vi "Popup Dialog.vi"(5 "Tab Control":T1, 8 "error in (no error)":errorcluster, 9 "show":bool, 10 "Error MSG":string, 11 "Delay (5sec)":dbl=5.0) -> (0 "error out":errorcluster, 1 "canceled?":bool, 3 "Answer MSG":string)   [LabVIEW 2020, in "Popup Dialog.lvlib"]
uses:
  Popup Dialog.lvlib
  Popup Dialog States.ctl
panel:
  in  "Complete MSG2":string="Press OK When Ready"
  in  "Complete MSG":string
  in  "Complete OK":bool
  in  "Fail OK":bool
  in  "Fail MSG":string
  in  "Prepare OK":bool
  in  "Stopping OK":bool
  in  "Error Try":bool
  in  "Error Break":bool
  out "Description:":string
  out "code":i32
  in  "Error Continue":bool
  in  "Saved OK":bool
  in  "Cancel":bool
  in  "Close OK":bool
  # "Complete"
  # "Preparing Test"
  # "Stopping Test..."
  # "There was an Error"
  # "Tests Saved"
  # "Saving"
  # "Please Wait..."
  # "Are you sure?"
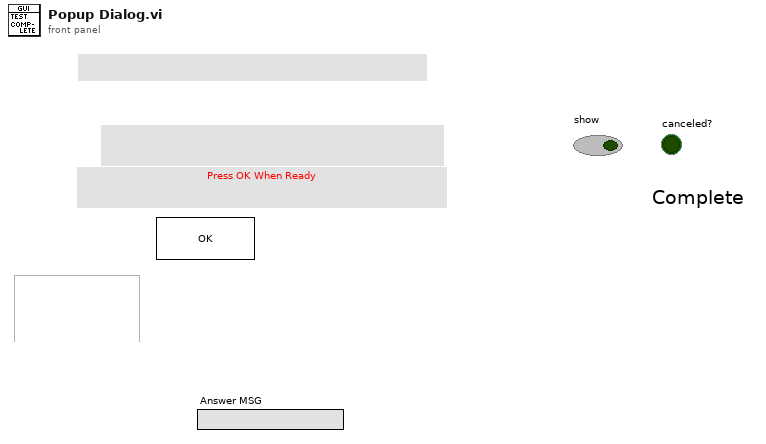
[diagram p1: front panel]
types:
  T1 = typedef "Popup Dialog.lvlib/Popup Dialog States.ctl" = enum32{"Complete", "Failed", "Preparing", "Stopping", "Error", "Saved", "Saving", "Closing"}
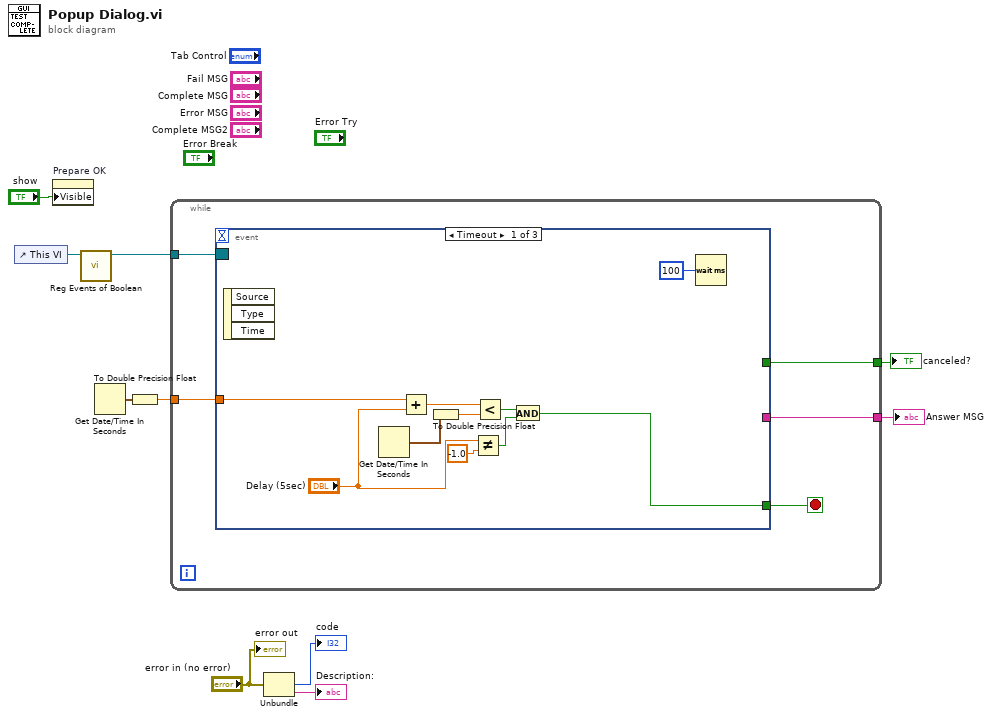
[diagram p0: block diagram]
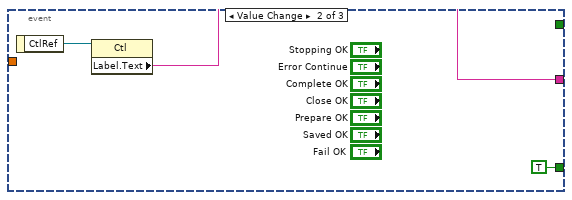
[diagram p2: hidden frame]
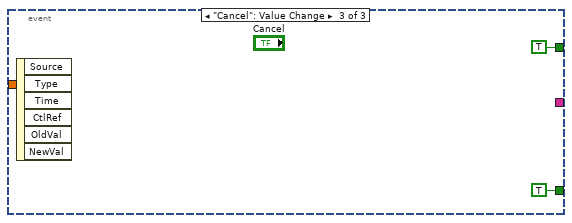
[diagram p3: hidden frame]
diagram:
  n1 = control-ref of="This VI"() -> (w4:refnum<vi>)
  n2 = property on="Prepare OK" class="Bool"("Visible"="show") -> ()  [unwired: 2 in, 2 out]
  n3 = call "Reg Events of Boolean.vi"("VI in"=w4) -> ("Event Registration Refnum out"=w3:refnum<event-registration>)  [unwired: 10 in]
  n4 = Get Date/Time In Seconds() -> (seconds since 1Jan1904=w6:timestamp)
  n5 = To Double Precision Float(number=w6) -> (double precision float=w5:dbl)
  n6 = while {
    tunnel: w5 -> [w15]
    tunnel: w3 -> [w13]
    tunnel: [w12] -> w2
    tunnel: [w11] -> w1
    stop <- w14 stop-if-true
    n7 = event shown="[0] Timeout" {
      selector: w13 -> [_ _ _]
      dyn-events: _ -> [_ _ _]
      timeout: _ -> [_ _ _]
      tunnel: w15 -> [w19 _ _]
      tunnel: [w17 TRUE TRUE] -> w14
      tunnel: [_ _ TRUE ("Cancel")] -> w12
      tunnel: [_ w26 _] -> w11
      event Timeout {
        n8 = event-data() -> ()  [unwired: 1 in, 3 out]
        n9 = Get Date/Time In Seconds() -> (seconds since 1Jan1904=w21:timestamp)
        n10 = Add(x=w19, y="Delay (5sec)") -> (x+y=w20:dbl)
        n11 = To Double Precision Float(number=w21) -> (double precision float=w18:dbl)
        n12 = Not Equal?(x="Delay (5sec)", y=-1.0) -> (x != y?=w25:bool)
        n13 = Less?(x=w20, y=w18) -> (x < y?=w24:bool)
        n14 = And(x=w24, y=w25) -> (x .and. y?=w17:bool)
        n15 = Wait (ms)(milliseconds to wait=u32 100) -> ()  [unwired: 1 out]
      }
      event Value Change {
        n16 = event-data() -> ("CtlRef"=w28:refnum<vi>)  [unwired: 1 in]
        n17 = property class="Ctl"(reference=w28) -> ("Label.Text"=w26:string)  [unwired: 1 in, 2 out]
      }
      event "Cancel": Value Change {
        n18 = event-data() -> ()  [unwired: 1 in, 6 out]
      }
    }
  }
  "canceled?" <- w2
  "Answer MSG" <- w1
  n19 = Unbundle("error in (no error)") -> ("code"=→"code":i32, "source"=→"Description:":string)  [unwired: 1 out]
  "error out" <- "error in (no error)"
